vi "NFC test.vi"() -> ()   [LabVIEW 2018]
panel:
  out "error out":errorcluster
  out "return value":string
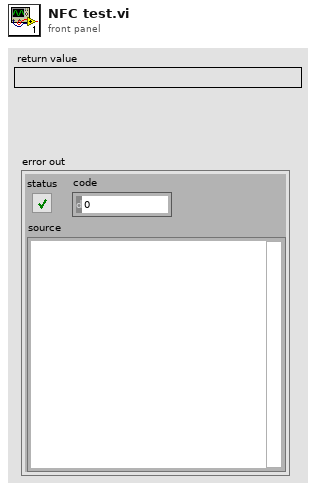
[diagram p1: front panel]
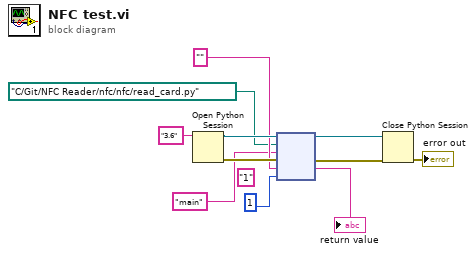
[diagram p0: block diagram]
diagram:
  (unwired) "1" ("Python version")
  n1 = Open Python Session(python version="3.6" ("Python version")) -> (session out=w10:refnum<k35>, error out=w7:errorcluster)  [unwired: 2 in]
  n2 = node(w10, path "C:/Git/NFC Reader/nfc/nfc/read_card.py" ("module path"), "main" ("function name"), w7, "" ("Python version"), 1) -> (w9:refnum<k35>, w8:errorcluster, →"return value":string)  [unwired: 1 in, 2 out]
  n3 = Close Python Session(session in=w9, error in=w8) -> (11:→"error out":errorcluster)
